vi "Global - Hold.vi"() -> ()   [LabVIEW 2019]
panel:
  in  "VISA Ref":refnum<visa-resource-name>
  in  "Data Unit":T1
  in  "error out":errorcluster
  out "Array":bool[](array[boolean])
  in  "Hold":bool
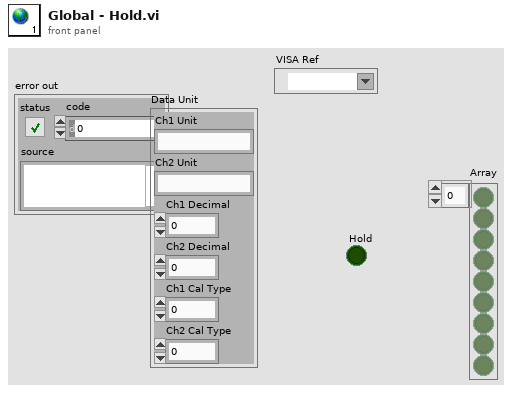
[diagram p1: front panel]
types:
  T1 = cluster{"Ch1 Unit":string, "Ch2 Unit":string, "Ch1 Decimal":u8, "Ch2 Decimal":u8, "Ch1 Cal Type":u8, "Ch2 Cal Type":u8}
diagram:
